vi "(SubVI) Cut Each Sections For pFC_YCC.vi"(0 "xDNA":dbl[](array[numeric]), 1 "Initial guess locations":i32[](array[numeric]), 2 "Diff (i-i+1)":dbl[](array[numeric]), 3 "Data Rate (Hz)":dbl, 4 "threshold y":dbl, 5 "# of adjencent points":i32=10) -> (6 "Total Peak location (index)":i32[](array[numeric]), 7 "Each Section First and End index":i32[](array[numeric]))   [LabVIEW 2014]
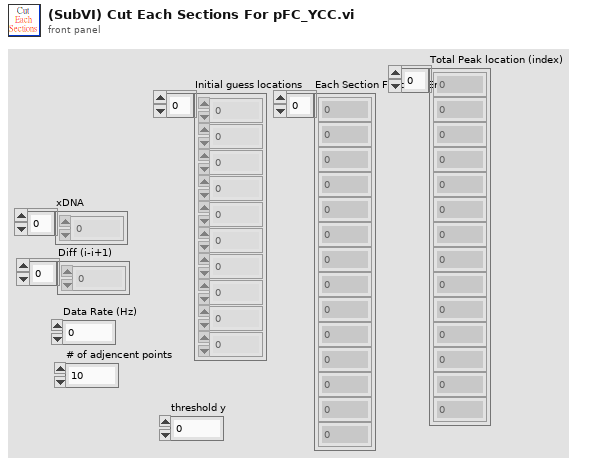
[diagram p1: front panel]
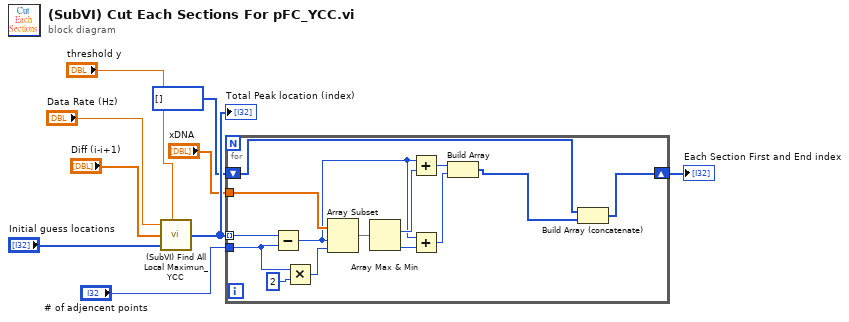
[diagram p0: block diagram]
diagram:
  n1 = call "(SubVI) Find All Local Maximun_YCC.vi"("Data Rate (Hz)"="Data Rate (Hz)", "threshold y"="threshold y", "Signal"="Diff (i-i+1)", "Initial guess locations"="Initial guess locations") -> ("Total Peak location (index)"=w6:i32[])  [unwired: 2 in, 1 out]
  "Total Peak location (index)" <- w6
  n2 = for {
    tunnel: w6 -> [w22] mode=indexing
    tunnel: "xDNA" -> [w23]
    tunnel: "# of adjencent points" -> [w20]
    shift-right: [w10] -> w2
    shift-left: i32[] [] -> [w12]
    n3 = Subtract(x=w22, y=w20) -> (x-y=w16:i32)
    n4 = Multiply(x=w20, y=2) -> (x*y=w19:i32)
    n5 = Array Subset(array=w23, index=w16, length=w19) -> (w18:dbl[])
    n6 = Array Max & Min(array=w18) -> (max index (indices)=w17:i32, min index (indices)=w15:i32)  [unwired: 2 out]
    n7 = Add(x=w16, y=w17) -> (x+y=w14:i32)
    n8 = Add(x=w16, y=w15) -> (x+y=w13:i32)
    n9 = Build Array(w14, w13) -> (w11:i32[])
    n10 = Build Array (concatenate)(w12, w11) -> (w10:i32[])
  }
  "Each Section First and End index" <- w2
